vi "PE Set Wavelength On Grating.vi"(8 "error in (no error)":errorcluster, 9 "wavelength":dbl, 10 "gratingIndex":i32, 11 "peHandle":u64) -> (0 "error out":errorcluster)   [LabVIEW 2015, in "PE_Filter_SDK.lvlib"]
doc: "PEFILTERSDK_API PE_STATUS PE_SetWavelengthOnGrating(PE_HANDLE peHandle, int gratingIndex, double wavelength);"
uses:
  PE_Filter_SDK.lvlib
  Documents/test/SDK 1.2.4 Installer/SDK 1.2.4 Installer/win64/PE_Filter_SDK.dll
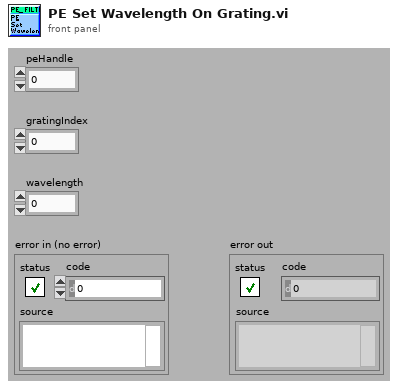
[diagram p1: front panel]
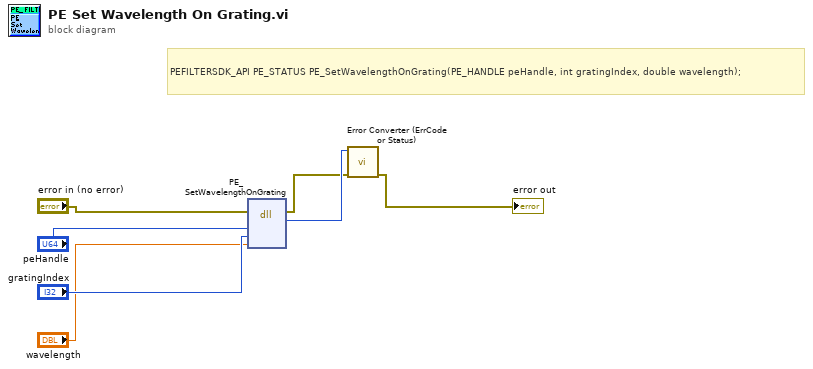
[diagram p0: block diagram]
diagram:
  # "PEFILTERSDK_API PE_STATUS PE_SetWavelengthOnGrating(PE_HANDLE peHandle, int gratingIndex, double wavelength);"
  n1 = dll-call lib="C:/Users/localAdmin/Documents/test/SDK 1.2.4 Installer/SDK 1.2.4 Installer/win64/PE_Filter_SDK.*" fn="PE_SetWavelengthOnGrating"(error in="error in (no error)", "peHandle"="peHandle", "gratingIndex"="gratingIndex", "wavelength"="wavelength") -> (error out=w2:errorcluster, "return type"=w3:i32)  [unwired: 5 in, 1 out]
  n2 = call "Error Converter (ErrCode or Status).vi"("error in (no error)"=w2, "error code"=w3) -> ("error out"=→"error out":errorcluster)  [unwired: 9 in]
